vi "ReadConnection.vi"(8 "error in (no error)":errorcluster, 11 "XPath expression":string="/LIST_OF_CONNECTIONS") -> (0 "error out":errorcluster, 1 "LastUpdated":timestamp format="%<%b %d %Y %H:%M:%S>T\n", 2 "path":path, 3 "ConnectionStatus":string, 5 "id":string)   [LabVIEW 2017]
uses:
  <vilib>/xml/Load XML File.vi
  <vilib>/xml/Close Reference(Node).vi
  <vilib>/xml/NI_XML.lvlib
  <resource>/objmgr/DOMUserDefRef.rc
panel:
  out "parse errors":string
  out "XML":string
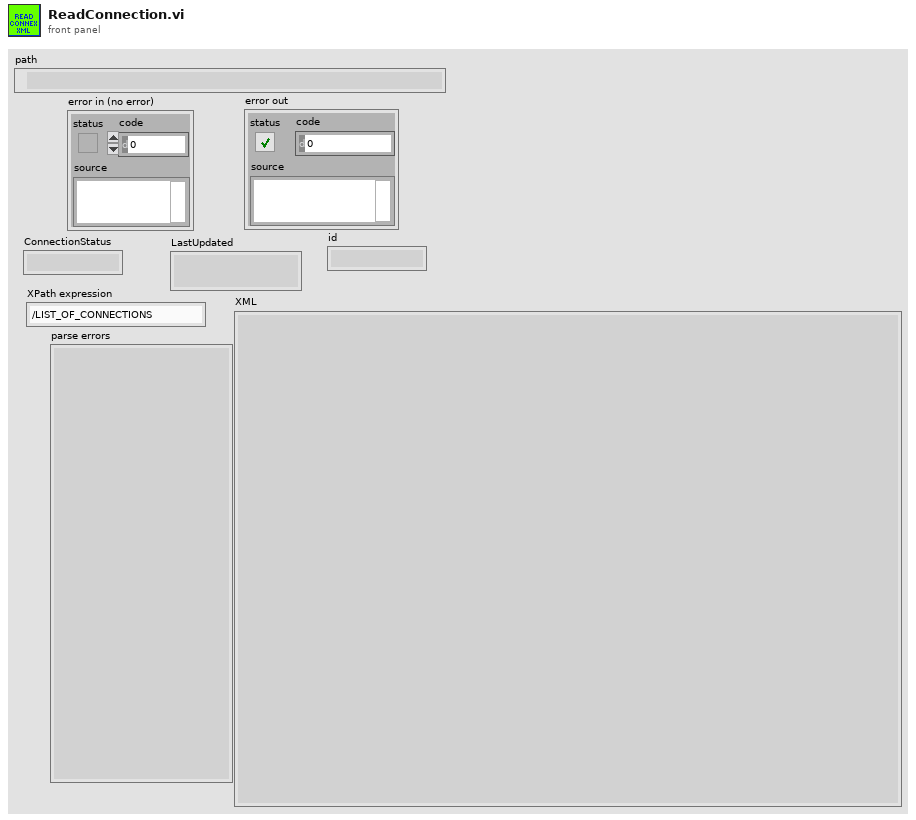
[diagram p1: front panel]
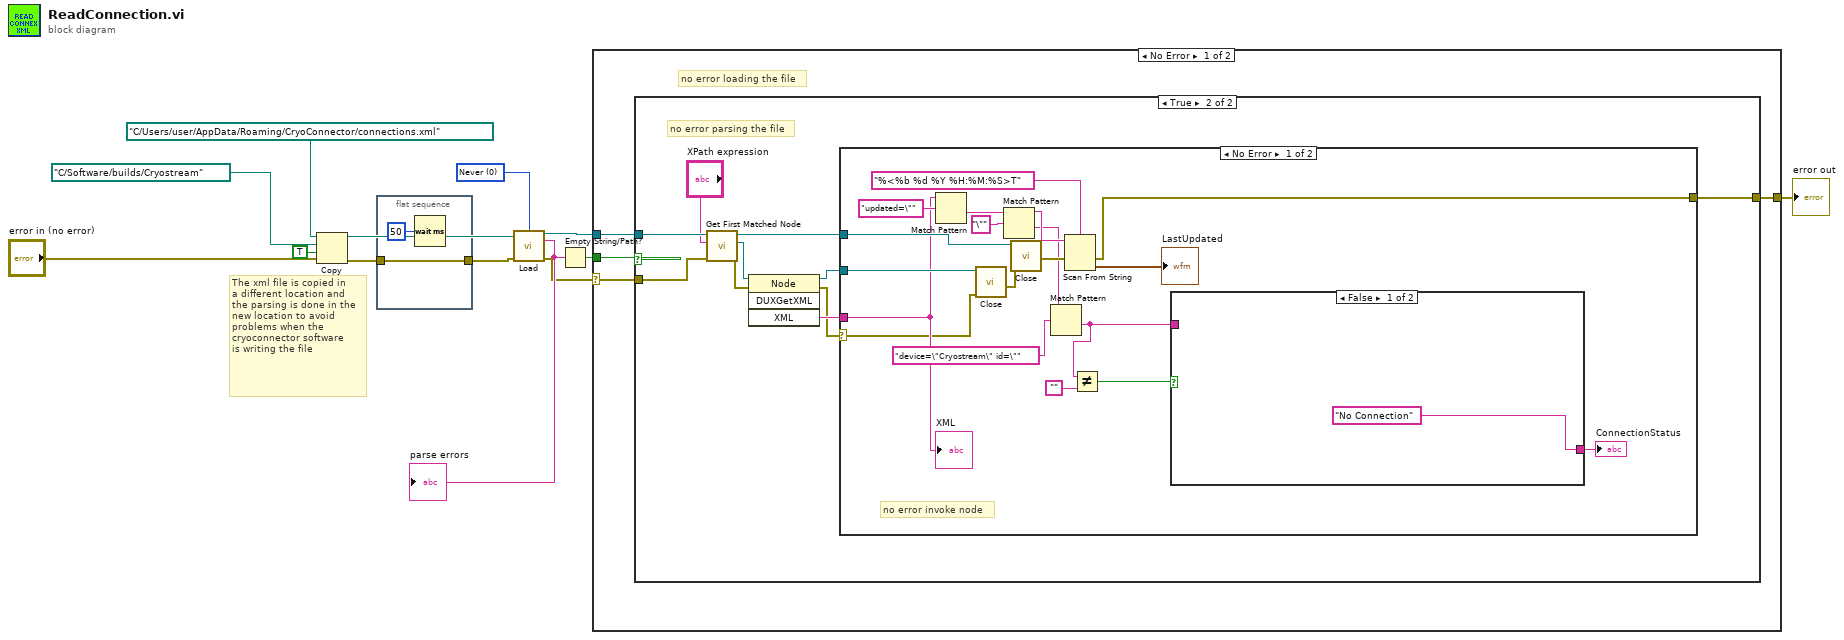
[diagram p0: block diagram]
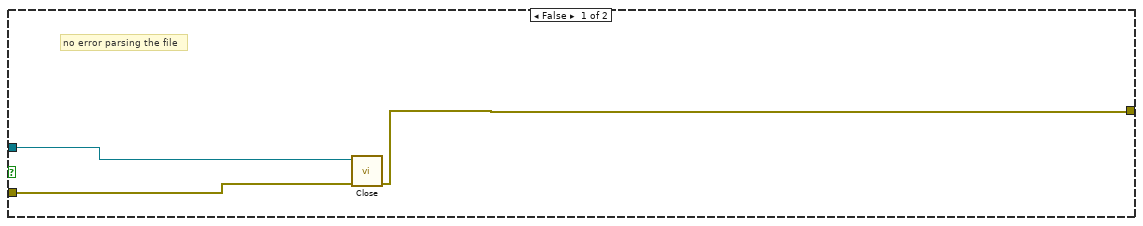
[diagram p2: hidden frame]
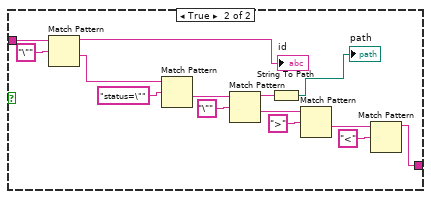
[diagram p3: hidden frame]
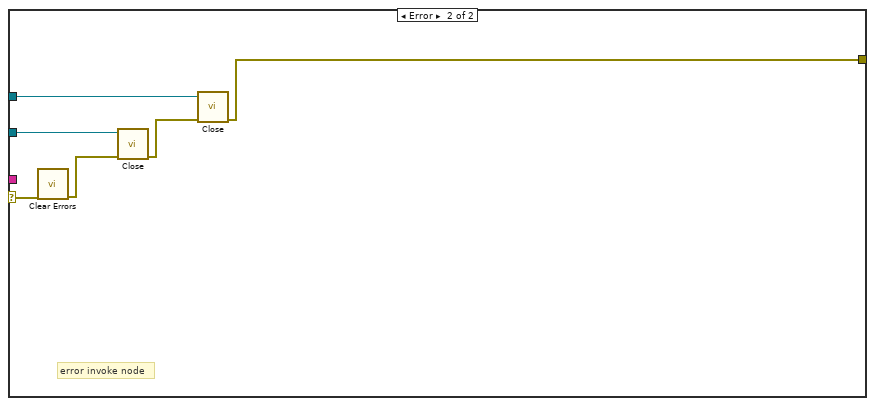
[diagram p4: hidden frame]
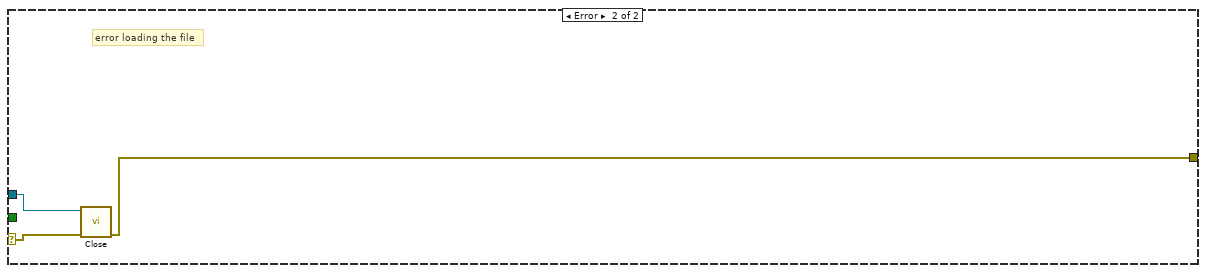
[diagram p5: hidden frame]
diagram:
  w8 = 0 items=["Never", "Always", "Auto"] ("validate on load (Auto)")
  # "The xml file is copied in\na different location and \nthe parsing is done in the\nnew location to avoid \nproblems when the \ncryoconnector software\nis writing the file"
  n1 = Copy(8:"error in (no error)", 9:TRUE ("overwrite (F)"), 10:path "C:/Software/builds/Cryostream" ("target path (use dialog)"), 11:path "C:/Users/user/AppData/Roaming/CryoConnector/connections.xml") -> (0:w3:errorcluster, 3:w1:path)  [unwired: 1 in, 1 out]
  n2 = flat-sequence {
    tunnel: w3 -> [w14]
    tunnel: [w14] -> w2
    frame #0 {
      n3 = Wait (ms)(milliseconds to wait=u32 50) -> ()  [unwired: 1 out]
    }
  }
  n4 = call-poly <vilib>:"Load.vi"("path to XML document"=w1, "validate on load (Auto)"=w8, "error in (no error)"=w2) -> ("DOM document out"=w13:refnum<k20>, "parse errors"=w11:string, "error out"=w9:errorcluster)  [unwired: 10 in]
  "parse errors" <- w11
  n5 = Empty String/Path?(string/path=w11) -> (empty?=w10:bool)
  n6 = case shown="No Error" w9 {
    selector: w9 -> [w16 w75]
    tunnel: w13 -> [w19 w74]
    tunnel: [w18 w73] -> w12
    tunnel: w10 -> [w17 _]
    frame No Error {
      # "no error loading the file"
      n7 = case shown="True" w17 {
        tunnel: w19 -> [w22 w32]
        tunnel: [w21 w31] -> w18
        tunnel: w16 -> [w20 w24]
        frame False {
          # "no error parsing the file"
          n8 = call-poly <vilib>:"Close.vi"("error in (no error)"=w20, "node"=w22) -> ("error out"=w21:errorcluster)  [unwired: 7 in]
        }
        frame True {
          # "no error parsing the file"
          n9 = call <vilib>:"Get First Matched Node.vi"("error in (no error)"=w24, "XPath expression"="XPath expression", "node in"=w32) -> ("error out"=w25:errorcluster, "node result"=w29:refnum<k20>, "node out"=w28:refnum<k20>)  [unwired: 6 in]
          n10 = invoke class="Node" method="DUXGetXML"(reference=w29, error in=w25) -> (reference out=w27:refnum<k20>, error out=w23:errorcluster, "XML"=w26:string)  [unwired: 2 in, 1 out]
          n11 = case shown="No Error" w23 {
            selector: w23 -> [w34 w68]
            tunnel: [w51 w69] -> w31
            tunnel: w28 -> [w39 w72]
            tunnel: w27 -> [w38 w71]
            tunnel: w26 -> [w35 _]
            frame No Error {
              # "no error invoke node"
              n12 = Match Pattern(string=w35, regular expression="updated=\"") -> (after substring=w48:string)  [unwired: 1 in, 3 out]
              n13 = call-poly <vilib>:"Close.vi"("error in (no error)"=w34, "node"=w38) -> ("error out"=w37:errorcluster)  [unwired: 7 in]
              n14 = Match Pattern(string=w48, regular expression="\"") -> (before substring=w44:string, after substring=w36:string)  [unwired: 1 in, 2 out]
              n15 = call-poly <vilib>:"Close.vi"("error in (no error)"=w37, "node"=w39) -> ("error out"=w40:errorcluster)  [unwired: 7 in]
              n16 = Match Pattern(string=w36, regular expression="device=\"Cryostream\" id=\"") -> (after substring=w42:string)  [unwired: 1 in, 3 out]
              n17 = Scan From String(format string="%<%b %d %Y %H:%M:%S>T", input string=w44, error in=w40) -> (error out=w51:errorcluster, output 1=→"LastUpdated":timestamp)  [unwired: 2 in, 2 out]
              n18 = Not Equal?(x=w42, y="") -> (x != y?=w43:bool)
              n19 = case shown="False" w43 {
                tunnel: w42 -> [_ w59]
                tunnel: ["No Connection" ("ConnectionStatus") w53] -> w33
                frame False {
                }
                frame True {
                  n20 = Match Pattern(string=w59, regular expression="\"") -> (before substring=→"id":string, after substring=w56:string)  [unwired: 1 in, 2 out]
                  n21 = Match Pattern(string=w56, regular expression="status=\"") -> (after substring=w58:string)  [unwired: 1 in, 3 out]
                  n22 = Match Pattern(string=w58, regular expression="\"") -> (before substring=w64:string, after substring=w57:string)  [unwired: 1 in, 2 out]
                  n23 = String To Path(string=w64) -> (path=→"path":path)
                  n24 = Match Pattern(string=w57, regular expression=">") -> (after substring=w61:string)  [unwired: 1 in, 3 out]
                  n25 = Match Pattern(string=w61, regular expression="<") -> (before substring=w53:string)  [unwired: 1 in, 3 out]
                }
              }
              "ConnectionStatus" <- w33
              "XML" <- w35
            }
            frame Error {
              # "error invoke node"
              n26 = call <vilib>:"Clear Errors.vi"("error in (no error)"=w68) -> ("error out"=w67:errorcluster)  [unwired: 5 in, 1 out]
              n27 = call-poly <vilib>:"Close.vi"("error in (no error)"=w67, "node"=w71) -> ("error out"=w70:errorcluster)  [unwired: 7 in]
              n28 = call-poly <vilib>:"Close.vi"("error in (no error)"=w70, "node"=w72) -> ("error out"=w69:errorcluster)  [unwired: 7 in]
            }
          }
        }
      }
    }
    frame Error {
      # "error loading the file"
      n29 = call-poly <vilib>:"Close.vi"("error in (no error)"=w75, "node"=w74) -> ("error out"=w73:errorcluster)  [unwired: 7 in]
    }
  }
  "error out" <- w12
